vi "Actor Core.vi"(8 "error in":errorcluster, 11 "Nested in":refnum<class "MQTT_Server_Actor.lvclass">) -> (0 "error out":errorcluster, 3 "Actor out":refnum<class "Actor.lvclass">)   [LabVIEW 2018, in "MQTT_Server_Actor.lvlib" / "MQTT_Server_Actor.lvclass"]
doc: "(<B>Filename</B>: Actor Framework.lvlib:Actor.lvclass:Actor Core.vi)\n\nReceives messages to the actor, reacts to them, and initiates any error handling that may shut the actor down.\n\nDescendant classes may override this VI to append parallel tasks for the actor to complete while it handles messages. Overrides use the Call Parent Method node."
uses:
  MQTT_Server_Actor.lvclass
  D:/Program Files (x86)/National Instruments/LabVIEW 2018/vi.lib/ActorFramework/Actor/Actor.lvclass
  <vilib>/ActorFramework/Actor/Actor.lvclass
  <vilib>/G Open Source Project for LabVIEW/MQTT Broker/Server class/Server.lvclass
  D:/Program Files (x86)/National Instruments/LabVIEW 2018/vi.lib/LabVIEW Open Source Project/MQTT Connection/MQTT_Base/Base Class/MQTT_Base.lvclass
  MQTT_Server_Actor.lvclass/MQTT_Server_Actor.ctl
  <vilib>/ActorFramework/Actor/Actor.lvclass/Actor.ctl
  <vilib>/ActorFramework/Message Enqueuer/Message Enqueuer.lvclass/Message Enqueuer.ctl
  <vilib>/LabVIEW Open Source Project/MQTT Connection/MQTT_Base/Base Class/MQTT_Base.lvclass/MQTT_Base.ctl
  <vilib>/G Open Source Project for LabVIEW/MQTT Broker/Server class/Server.lvclass/Server.ctl
  <vilib>/LabVIEW Open Source Project/MQTT Control Packets/Control Packets/ControlPacket/ControlPacket.lvclass/ControlPacket.ctl
  <vilib>/G Open Source Project for LabVIEW/MQTT Broker/PacketTracer/PacketTracer.lvclass
  <vilib>/ActorFramework/Message Enqueuer/Init from Existing Queue.vi
  <vilib>/ActorFramework/Message Enqueuer/Enqueue.vi
  <vilib>/ActorFramework/Stop Msg/Stop Msg.lvclass
  D:/Program Files (x86)/National Instruments/LabVIEW 2018/vi.lib/ActorFramework/Message/Message.lvclass
  <vilib>/LabVIEW Open Source Project/MQTT Control Packets/Control Packets/PUBLISH/PUBLISH.lvclass
  D:/Program Files (x86)/National Instruments/LabVIEW 2018/vi.lib/LabVIEW Open Source Project/MQTT Control Packets/Control Packets/ControlPacket/ControlPacket.lvclass
  <vilib>/LabVIEW Open Source Project/Connection/Connection.TCP/Connection.TCP.lvclass
  D:/Program Files (x86)/National Instruments/LabVIEW 2018/vi.lib/LabVIEW Open Source Project/Connection/Connection/Connection.lvclass
  <vilib>/ActorFramework/Message Priority Queue/Priority Enqueue.vi
  <vilib>/ActorFramework/Message Enqueuer/Message Enqueuer.lvclass
  <vilib>/LabVIEW Open Source Project/MQTT Control Packets/Control Packets/ControlPacket/ControlPacket.lvclass
  <vilib>/LabVIEW Open Source Project/MQTT Connection/MQTT_Base/Base Class/MQTT_Base.lvclass
  MQTT_Server_Actor Messages/1_StartStopServer Msg/1_StartStopServer Msg.lvclass
panel:
  in  "Port":u16=1883
  out "Broker":string
  out "字符串":string
  out "Active?":bool
  in  "StartStop":enum32{"START", "STOP"}(radio)
  out "Clients":u32
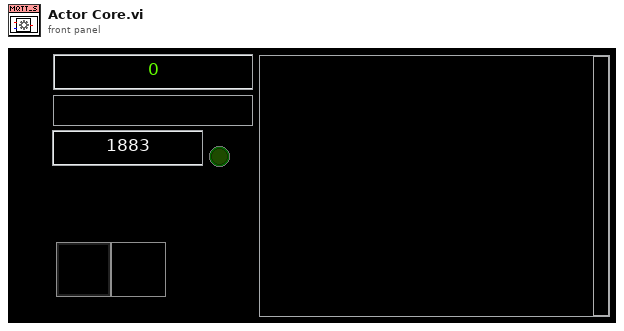
[diagram p1: front panel]
types:
  T1 = cluster{"Stop":refnum<user-event>, "StartServer":refnum<user-event>}
  T2 = typedef "MQTT Base.lvlib/MQTT_Base.lvclass/Public Events -- cluster.ctl" = cluster{"Stop Event":refnum<user-event>, "Error Event":refnum<user-event>, "Inbound Message":refnum<user-event>}
  T3 = typedef "MQTT Server.lvlib/Server.lvclass/Public Events -- cluster.ctl" = cluster{"NbConnections":refnum<user-event>, "Client Event":refnum<user-event>}
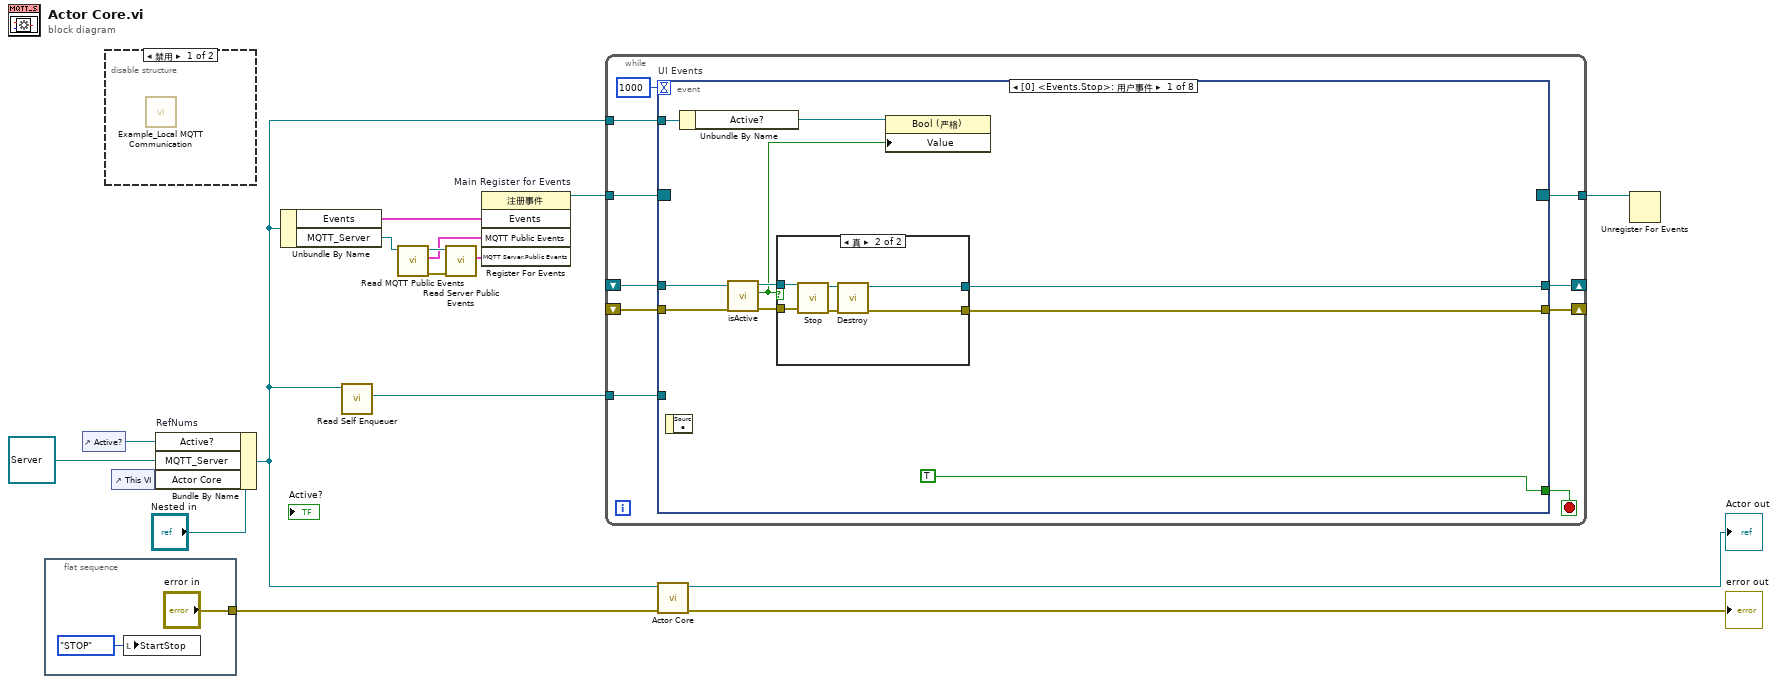
[diagram p0: block diagram]
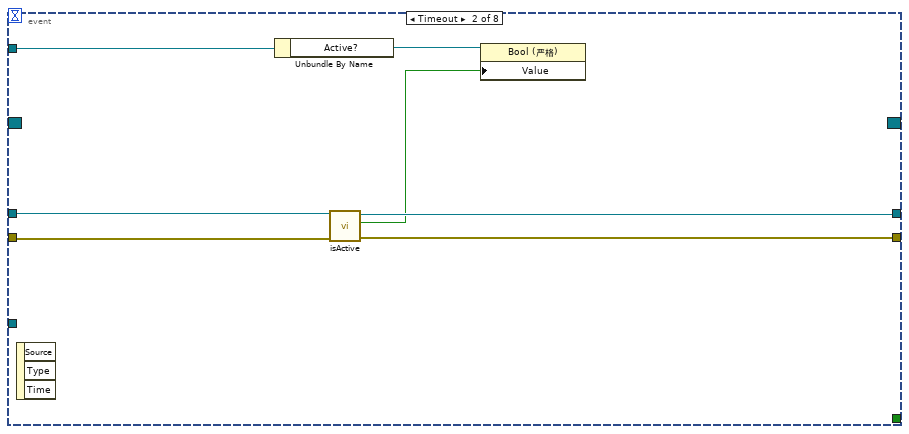
[diagram p4: hidden frame]
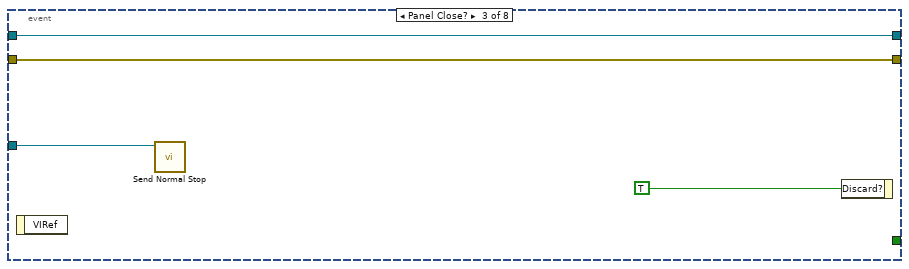
[diagram p5: hidden frame]
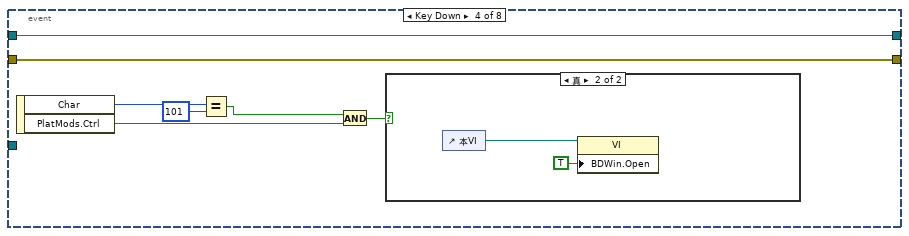
[diagram p6: hidden frame]
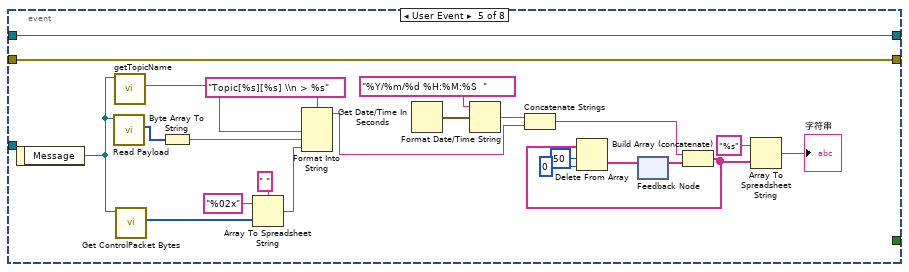
[diagram p8: hidden frame]
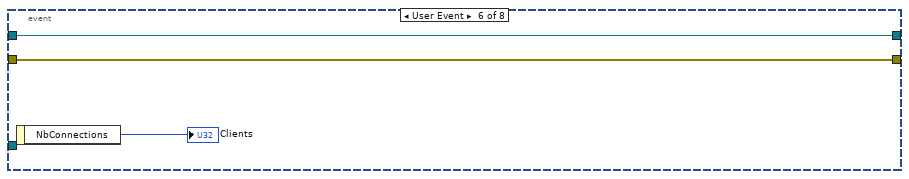
[diagram p9: hidden frame]
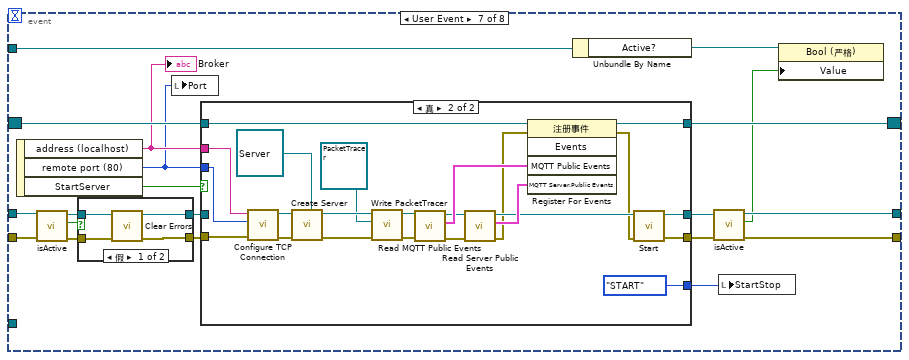
[diagram p10: hidden frame]
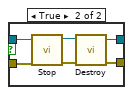
[diagram p11: hidden frame]
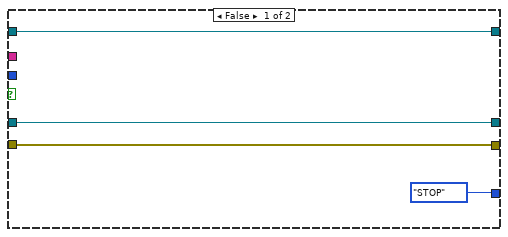
[diagram p12: hidden frame]
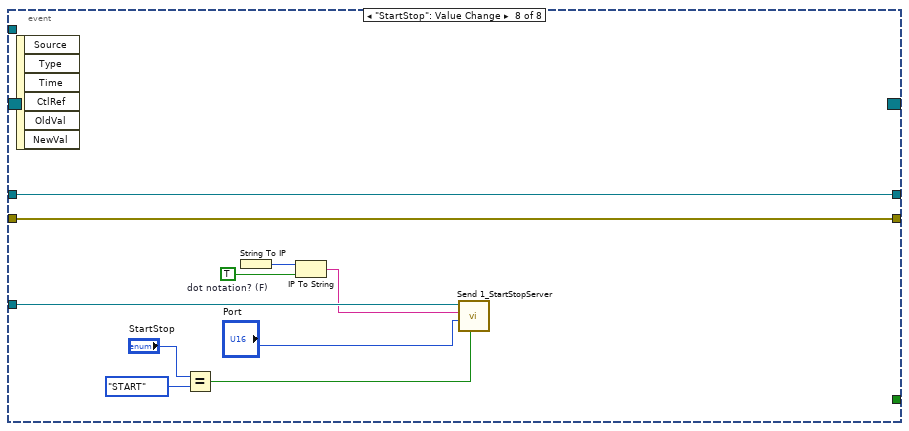
[diagram p13: hidden frame]
diagram:
  n1 = flat-sequence {
    tunnel: ["error in"] -> w9
    frame #0 {
      n2 = local write "StartStop"(enum32{"START", "STOP"}."STOP" ("StartStop")) -> ()
    }
  }
  n3 = control-ref of="Active?"() -> (w2:refnum<vi>)
  n4 = disable-structure shown="禁用" {
    frame Disabled {
      n5 = call <vilib>:"Example_Local MQTT Communication.vi"() -> ()  [unwired: 12 in]
    }
    frame Enabled {
    }
  }
  n6 = control-ref of="This VI"() -> (w10:refnum<vi>)
  n7 = Bundle By Name "RefNums"(cluster="Nested in", "Active?"=w2, "MQTT_Server"=refnum<class "Server.lvclass"> refnum, "Actor Core"=w10) -> (w1:refnum<class "MQTT_Server_Actor.lvclass">)
  n8 = Unbundle By Name(w1) -> ("Events"=w14:T1, "MQTT_Server"=w5:refnum<class "Server.lvclass">)
  n9 = call <vilib>:"Read Self Enqueuer.vi"("Actor"=w1) -> ("Self Enqueuer"=w12:refnum<class "Message Enqueuer.lvclass">)  [unwired: 10 in]
  n10 = call <vilib>:"Read MQTT Public Events.vi"("MQTT_Base in"=w5) -> ("error out"=w6:errorcluster, "MQTT Public Events"=w4:T2, "MQTT_Base out"=w7:refnum<class "Server.lvclass">)  [unwired: 8 in]
  n11 = call <vilib>:"Read Server Public Events.vi"("error in (no error)"=w6, "Server in"=w7) -> ("MQTT Server.Public Events"=w3:T3)  [unwired: 7 in, 2 out]
  n12 = register-events "Main Register for Events"(w14, w4, w3) -> (reference out=w15:refnum<event-registration>)  [unwired: 2 in, 1 out]
  n13 = while {
    tunnel: w15 -> [w29]
    tunnel: [w27] -> w13
    tunnel: w12 -> [w26]
    shift-right: [w24] -> _
    shift-left: _ -> [w22]
    shift-right: [w25] -> _
    shift-left: _ -> [w23]
    tunnel: w1 -> [w20]
    stop <- w28 stop-if-true
    n14 = event "UI Events" shown="[0] <Events.Stop>: 用户事件" {
      selector: w29 -> [_ _ _ _ _ _ w113 _]
      dyn-events: [_ _ _ _ _ _ w112 _] -> w27
      timeout: 1000 -> [_ _ _ _ _ _ _ _]
      tunnel: [TRUE _ _ _ _ _ _ _] -> w28
      tunnel: w26 -> [_ _ w57 _ _ _ _ w157]
      tunnel: [w38 w54 w56 w65 w90 w92 w107 w159] -> w25
      tunnel: [w37 w53 w55 w64 w89 w91 w106 w158] -> w24
      tunnel: w23 -> [w36 w52 w56 w65 w90 w92 w105 w159]
      tunnel: w22 -> [w35 w51 w55 w64 w89 w91 w104 w158]
      tunnel: w20 -> [w31 w50 _ _ _ _ w98 _]
      event User Event {
        n15 = event-data() -> ()  [unwired: 1 in, 1 out]
        n16 = Unbundle By Name(w31) -> ("Active?"=w32:refnum<vi>)
        n17 = call <vilib>:"isActive.vi"("error in (no error)"=w35, "MQTT_Base in"=w36) -> ("error out"=w33:errorcluster, "Active?"=w30:bool, "MQTT_Base out"=w34:refnum<class "MQTT_Base.lvclass">)  [unwired: 7 in]
        n18 = case shown="真" w30 {
          tunnel: [w41 w45] -> w38
          tunnel: [w40 w44] -> w37
          tunnel: w34 -> [w41 w43]
          tunnel: w33 -> [w40 w42]
          frame False {
          }
          frame True {
            n19 = call <vilib>:"Stop.vi"("error in (no error)"=w42, "MQTT_Base in"=w43) -> ("error out"=w47:errorcluster, "MQTT_Base out"=w46:refnum<class "MQTT_Base.lvclass">)  [unwired: 7 in, 1 out]
            n20 = call <vilib>:"Destroy.vi"("error in (no error)"=w47, "MQTT_Base in"=w46) -> ("error out"=w44:errorcluster, "MQTT_Base out"=w45:refnum<class "MQTT_Base.lvclass">)  [unwired: 8 in]
          }
        }
        n21 = property class="Bool (严格)"(reference=w32, "Value"=w30) -> ()  [unwired: 1 in, 2 out]
      }
      event Timeout {
        n22 = event-data() -> ()  [unwired: 1 in, 3 out]
        n23 = Unbundle By Name(w50) -> ("Active?"=w49:refnum<vi>)
        n24 = call <vilib>:"isActive.vi"("error in (no error)"=w51, "MQTT_Base in"=w52) -> ("error out"=w53:errorcluster, "Active?"=w48:bool, "MQTT_Base out"=w54:refnum<class "MQTT_Base.lvclass">)  [unwired: 7 in]
        n25 = property class="Bool (严格)"(reference=w49, "Value"=w48) -> ()  [unwired: 1 in, 2 out]
      }
      event Panel Close? {
        n26 = event-data() -> ()  [unwired: 1 in, 1 out]
        n27 = call <vilib>:"Send Normal Stop.vi"("Message Enqueuer"=w57) -> ()  [unwired: 10 in, 1 out]
        n28 = event-data("Discard?"=TRUE) -> ()  [unwired: 1 in, 1 out]
      }
      event Key Down {
        n29 = event-data() -> ("Char"=w63:i16, "PlatMods.Ctrl"=w60:bool)  [unwired: 1 in]
        n30 = Equal?(x=w63, y=i16 101) -> (x = y?=w61:bool)
        n31 = And(x=w61, y=w60) -> (x .and. y?=w59:bool)
        n32 = case shown="真" w59 {
          frame False {
          }
          frame True {
            n33 = control-ref of="本VI"() -> (w67:refnum<vi>)
            n34 = property class="VI"(reference=w67, "BDWin.Open"=TRUE ("程序框图窗口:打开")) -> ()  [unwired: 1 in, 2 out]
          }
        }
      }
      event User Event {
        n35 = event-data() -> ("Message"=w70:refnum<class "PUBLISH.lvclass">)  [unwired: 1 in]
        n36 = call <vilib>:"Read Payload.vi"("ControlPacket in"=w70) -> ("Payload"=w69:u8[])  [unwired: 9 in, 1 out]
        n37 = call <vilib>:"getTopicName.vi"("PUBLISH in"=w70) -> ("Topic"=w87:string)  [unwired: 8 in, 2 out]
        n38 = call <vilib>:"Get ControlPacket Bytes.vi"("ControlPacket"=w70) -> ("Bytes Stream"=w71:u8[])  [unwired: 7 in, 3 out]
        n39 = Byte Array To String(unsigned byte array=w69) -> (string=w68:string)
        n40 = Array To Spreadsheet String(delimiter (Tab)=" ", array=w71, 3:"%02x" ("format string")) -> (spreadsheet string=w88:string)
        n41 = Format Into String(format string="Topic[%s][%s] \\n > %s", w87, w68, w88) -> (resulting string=w75:string)  [unwired: 2 in, 1 out]
        n42 = Get Date/Time In Seconds() -> (seconds since 1Jan1904=w83:timestamp)
        n43 = Format Date/Time String(time format string (%c)="%Y/%m/%d %H:%M:%S  " ("时间格式字符串(%c)"), seconds (now)=w83) -> (date/time string=w82:string)  [unwired: 1 in]
        n44 = Concatenate Strings(w82, w75) -> (w80:string)
        n45 = feedback #1() -> (w79:string[])  [unwired: 1 in]
        n46 = Build Array (concatenate)(w80, w79) -> (w74:string[])
        n47 = Delete From Array(array=w74, length=50 ("长度"), index=0 ("索引")) -> (deleted portion=w76:string[])  [unwired: 1 out]
        n48 = feedback-in #1(w76) -> ()
        n49 = Array To Spreadsheet String(array=w74, 3:"%s" ("格式字符串")) -> (spreadsheet string=→"字符串":string)  [unwired: 1 in]
      }
      event User Event {
        n50 = event-data() -> ("NbConnections"=→"Clients":u32)  [unwired: 1 in]
      }
      event User Event {
        n51 = event-data() -> ("address (localhost)"=w95:string, "remote port (80)"=w94:u16, "StartServer"=w111:bool)  [unwired: 1 in]
        "Broker" <- w95
        n52 = call <vilib>:"isActive.vi"("error in (no error)"=w104, "MQTT_Base in"=w105) -> ("error out"=w100:errorcluster, "Active?"=w102:bool, "MQTT_Base out"=w101:refnum<class "MQTT_Base.lvclass">)  [unwired: 7 in]
        n53 = case shown="假" w102 {
          tunnel: [w116 w120] -> w110
          tunnel: [w114 w119] -> w103
          tunnel: w101 -> [w116 w118]
          tunnel: w100 -> [w115 w117]
          frame False {
            n54 = call <vilib>:"Clear Errors.vi"("error in (no error)"=w115) -> ("error out"=w114:errorcluster)  [unwired: 5 in, 1 out]
          }
          frame True {
            n55 = call <vilib>:"Stop.vi"("error in (no error)"=w117, "MQTT_Base in"=w118) -> ("error out"=w122:errorcluster, "MQTT_Base out"=w121:refnum<class "MQTT_Base.lvclass">)  [unwired: 7 in, 1 out]
            n56 = call <vilib>:"Destroy.vi"("error in (no error)"=w122, "MQTT_Base in"=w121) -> ("error out"=w119:errorcluster, "MQTT_Base out"=w120:refnum<class "MQTT_Base.lvclass">)  [unwired: 8 in]
          }
        }
        n57 = local write "Port"(w94) -> ()
        n58 = case shown="真" w111 {
          tunnel: w95 -> [_ w145]
          tunnel: w94 -> [_ w144]
          tunnel: w113 -> [w126 w142]
          tunnel: [w126 w141] -> w112
          tunnel: [w125 w133] -> w109
          tunnel: [w124 w132] -> w108
          tunnel: w103 -> [w124 w129]
          tunnel: w110 -> [w125 _]
          tunnel: [enum32{"START", "STOP"}."STOP" ("StartStop") enum32{"START", "STOP"}."START" ("StartStop")] -> w96
          frame False {
          }
          frame True {
            n59 = call <vilib>:"Configure TCP Connection.vi"("error in (no error)"=w129, "remote port (80)"=w144, "address (localhost)"=w145) -> ("error out"=w143:errorcluster, "Connection.TCP"=w146:refnum<class "Connection.TCP.lvclass">)  [unwired: 7 in]
            n60 = call <vilib>:"Create Server.vi"("Server in"=refnum<class "Server.lvclass"> refnum, "error in (no error)"=w143, "Connection Configuration"=w146) -> ("error out"=w148:errorcluster, "Server"=w149:refnum<class "Server.lvclass">)  [unwired: 7 in]
            n61 = call <vilib>:"Write PacketTracer.vi"("error in (no error)"=w148, "PacketTracer"=refnum<class "PacketTracer.lvclass"> refnum ("MQTT Server.lvlib:PacketTracer.lvclass"), "Server in"=w149) -> ("error out"=w140:errorcluster, "Server out"=w136:refnum<class "Server.lvclass">)  [unwired: 7 in]
            n62 = call <vilib>:"Read MQTT Public Events.vi"("error in (no error)"=w140, "MQTT_Base in"=w136) -> ("error out"=w135:errorcluster, "MQTT Public Events"=w139:T2, "MQTT_Base out"=w137:refnum<class "Server.lvclass">)  [unwired: 7 in]
            n63 = call <vilib>:"Read Server Public Events.vi"("error in (no error)"=w135, "Server in"=w137) -> ("error out"=w130:errorcluster, "MQTT Server.Public Events"=w138:T3, "Server out"=w134:refnum<class "Server.lvclass">)  [unwired: 7 in]
            n64 = register-events(reference=w142, error in=w130, w139, w138) -> (reference out=w141:refnum<event-registration>, error out=w131:errorcluster)  [unwired: 1 in]
            n65 = call <vilib>:"Start.vi"("error in (no error)"=w131, "MQTT_Base in"=w134) -> ("error out"=w132:errorcluster, "MQTT_Base out"=w133:refnum<class "Server.lvclass">)  [unwired: 7 in, 1 out]
          }
        }
        n66 = Unbundle By Name(w98) -> ("Active?"=w99:refnum<vi>)
        n67 = call <vilib>:"isActive.vi"("error in (no error)"=w108, "MQTT_Base in"=w109) -> ("error out"=w106:errorcluster, "Active?"=w97:bool, "MQTT_Base out"=w107:refnum<class "MQTT_Base.lvclass">)  [unwired: 7 in]
        n68 = local write "StartStop"(w96) -> ()
        n69 = property class="Bool (严格)"(reference=w99, "Value"=w97) -> ()  [unwired: 1 in, 2 out]
      }
      event "StartStop": Value Change {
        w152 = TRUE  # dot notation? (F)
        n70 = event-data() -> ()  [unwired: 1 in, 6 out]
        n71 = Equal?(x="StartStop", y=enum32{"START", "STOP"}."START") -> (x = y?=w154:bool)
        n72 = String To IP() -> (0:w153:u32)  [unwired: 1 in]
        n73 = IP To String(1:w152, 2:w153) -> (0:w151:string)
        n74 = call "Send 1_StartStopServer.vi"("T:start"=w154, "remote port (80)"="Port", "address (localhost)"=w151, "Message Enqueuer in"=w157) -> ()  [unwired: 6 in, 2 out]
      }
    }
  }
  n75 = call-parent "Actor Core.vi"("error in"=w9, "Actor in"=w1) -> ("error out"=→"error out":errorcluster, "Actor out"=→"Actor out":refnum<class "Actor.lvclass">)  [unwired: 8 in]
  n76 = Unregister For Events(event registration refnum=w13) -> ()  [unwired: 1 in, 1 out]
